vi "Get Time Stamp.vi"(8 "error in (no error)":errorcluster) -> (0 "error out":errorcluster, 1 "Seconds since 1Jan1904":timestamp)   [LabVIEW 2019, in "ProjectBuilder.lvlib"]
doc: "Error cluster synchronization for 'Get Date/Time in Seconds'."
uses:
  ProjectBuilder.lvlib
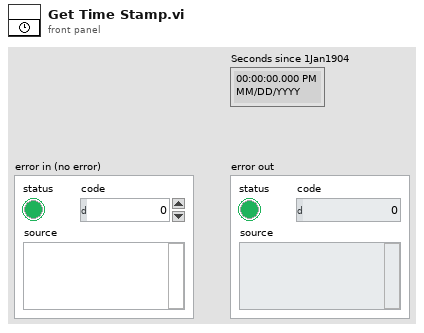
[diagram p1: front panel]
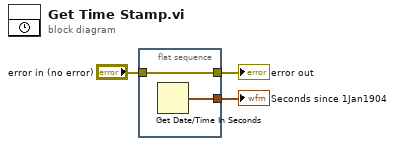
[diagram p0: block diagram]
diagram:
  n1 = flat-sequence {
    tunnel: [w5] -> w1
    tunnel: [w4] -> w2
    tunnel: "error in (no error)" -> [w4]
    frame #0 {
      n2 = Get Date/Time In Seconds() -> (seconds since 1Jan1904=w5:timestamp)
    }
  }
  "error out" <- w2
  "Seconds since 1Jan1904" <- w1
